vi "Climb Published Globals.vi"() -> ()   [LabVIEW 2018]
doc: "This is used primarily to publish values that other subsystems or user code may want to read periodically. It may also contain some settings such as debug switches or implementation selections that are independent of the operating mode of the subsystem."
uses:
  Climb Setpoints.ctl
  Climb Operations.ctl
  <vilib>/Rock Robotics/WPI/Framework/Command Status Info.ctl
  <vilib>/Rock Robotics/WPI/Framework/Completion Status.ctl
  <vilib>/Rock Robotics/WPI/Framework/Completion Notifier.ctl
panel:
  in  "Current Command":T6={"Current Command"={"Operation"=enum."Read Current", "Setpoint Rhino"=0.0, "Setpoint WHEELS"=0.0, "Roll"=0.0, "Pitch"=0.0, "Reset"=FALSE, "Speedy Tilt"={"Right"=TRUE, "Left"=TRUE}, "Climb"=enum."Level 1-3", "New Pos?"=FALSE, "Defense mode?"=FALSE}, "Command Timing"={"Start Time (ms)"=0, "Iterations"=0}, "Command Arguments"={"Command Info"={"Name"="", "Status"=enum."Successful", "notifier out"=refnum}, "Description"="", "Default Command"={"Operation"=enum."Read Current", "Setpoint Rhino"=0.0, "Setpoint WHEELS"=0.0, "Roll"=0.0, "Pitch"=0.0, "Reset"=FALSE, "Speedy Tilt"={"Right"=TRUE, "Left"=TRUE}, "Climb"=enum."Level 1-3", "New Pos?"=FALSE, "Defense mode?"=FALSE}, "queue out"=refnum, "Subsystem Name"=""}}
  # "Tip: The global is a good way publish state or\ninformational/debugging values.\nIt is not  advised that you put setpoint values here."
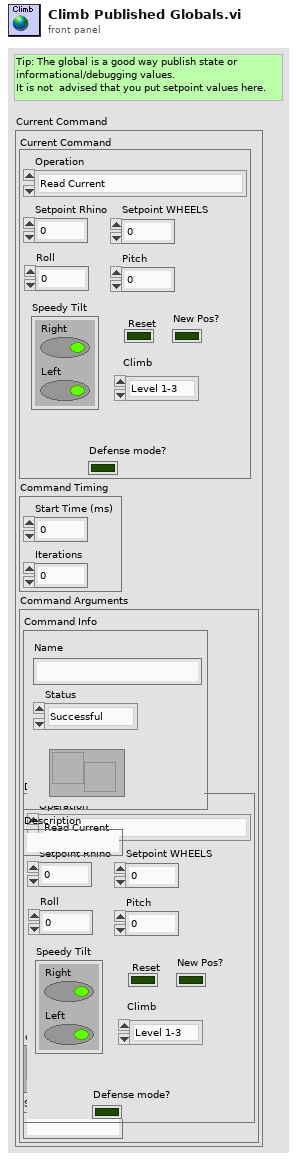
[diagram p1: front panel]
types:
  T1 = typedef "Climb Setpoints.ctl" = cluster{"Operation":T2, "Setpoint Rhino":dbl, "Setpoint WHEELS":dbl, "Roll":dbl, "Pitch":dbl, "Reset":bool, "Speedy Tilt":cluster{"Right":bool, "Left":bool}, "Climb":enum16{"Level 1-3", "Level 1-2", "Level 2-3"}, "New Pos?":bool, "Defense mode?":bool}
  T2 = typedef "Climb Operations.ctl" = enum16{"Reserve", "Read Current", "Immediate", "Ready", "Auto-Climb", "Reset/Turbo-Tilt", "Manual Climb"}
  T3 = typedef "Command Status Info.ctl" = cluster{"Name":string, "Status":T4, "notifier out":T5}
  T4 = typedef "Completion Status.ctl" = enum16{"Successful", "Aborted", "Incomplete"}
  T5 = typedef "Completion Notifier.ctl" = refnum<notifier>
  T6 = cluster{"Current Command":T1, "Command Timing":cluster{"Start Time (ms)":u32, "Iterations":i32}, "Command Arguments":cluster{"Command Info":T3, "Description":string, "Default Command":T1, "queue out":refnum<queue>, "Subsystem Name":string}}
diagram:
